vi "0x52.vi"(8 "error in":errorcluster, 10 "NTable":i32, 11 "paramUnicorn":T1={"conParam"={"ReadIntParam"=TRUE, "ReadDescrParam"=FALSE, "ReadFloatParam"=TRUE, "debug"=FALSE, "ReadJSON"=TRUE, "IP_address"="192.168.1.216", "N_attempts"=3, "type_con"=enum."TCP", "MB_address"=1, "VISA"="COM1", "connection ID"=refnum, "nameDevices"="", "timeout"=3000, "port"=2000, "type_version"="0F0C0001", "baud_rate"=115200, "VersionControl"=TRUE, "TCP_conn"=TRUE, "WindowSize"=700}, "Param"={"NumParam"={"NTelem"=201, "NInt"=16, "NFloat"=10, "NTable"=2}, "ParamInt"=[{"ID"="Режим работы", "Num"=0, "Name"="", "Type"="", "Enum"="", "Desc"="", "Unit"="", "Access"="", "FormatStr"="", "Min"=0, "Max"=0}, {"ID"="", "Num"=0, "Name"="", "Type"="", "Enum"="", "Desc"="", "Unit"="", "Access"="", "FormatStr"="", "Min"=0, "Max"=0}, {"ID"="", "Num"=0, "Name"="", "Type"="", "Enum"="", "Desc"="", "Unit"="", "Access"="", "FormatStr"="", "Min"=0, "Max"=0}, {"ID"="", "Num"=0, "Name"="", "Type"="", "Enum"="", "Desc"="", "Unit"="", "Access"="", "FormatStr"="", "Min"=0, "Max"=0}, {"ID"="", "Num"=0, "Name"="", "Type"="", "Enum"="", "Desc"="", "Unit"="", "Access"="", "FormatStr"="", "Min"=0, "Max"=0}, {"ID"="", "Num"=0, "Name"="", "Type"="", "Enum"="", "Desc"="", "Unit"="", "Access"="", "FormatStr"="", "Min"=0, "Max"=0}, {"ID"="ModeWork", "Num"=0, "Name"="", "Type"="", "Enum"="", "Desc"="", "Unit"="", "Access"="", "FormatStr"="", "Min"=0, "Max"=0}], "Telemetry"=[], "Table"=[], "ParamFloat"=[]}}) -> (0 "error out":errorcluster, 1 "ArrayFract32":fxp<+/-,32,1>[](array[numeric]), 2 "Table1D":sgl[](array[numeric]), 3 "paramUnicorn 2":T1={"conParam"={"ReadIntParam"=TRUE, "ReadDescrParam"=FALSE, "ReadFloatParam"=TRUE, "debug"=FALSE, "ReadJSON"=TRUE, "IP_address"="192.168.1.216", "N_attempts"=3, "type_con"=enum."TCP", "MB_address"=1, "VISA"="COM1", "connection ID"=refnum, "nameDevices"="", "timeout"=3000, "port"=2000, "type_version"="0F0C0001", "baud_rate"=115200, "VersionControl"=TRUE, "TCP_conn"=TRUE, "WindowSize"=700}, "Param"={"NumParam"={"NTelem"=201, "NInt"=16, "NFloat"=10, "NTable"=2}, "ParamInt"=[{"ID"="Режим работы", "Num"=0, "Name"="", "Type"="", "Enum"="", "Desc"="", "Unit"="", "Access"="", "FormatStr"="", "Min"=0, "Max"=0}, {"ID"="", "Num"=0, "Name"="", "Type"="", "Enum"="", "Desc"="", "Unit"="", "Access"="", "FormatStr"="", "Min"=0, "Max"=0}, {"ID"="", "Num"=0, "Name"="", "Type"="", "Enum"="", "Desc"="", "Unit"="", "Access"="", "FormatStr"="", "Min"=0, "Max"=0}, {"ID"="", "Num"=0, "Name"="", "Type"="", "Enum"="", "Desc"="", "Unit"="", "Access"="", "FormatStr"="", "Min"=0, "Max"=0}, {"ID"="", "Num"=0, "Name"="", "Type"="", "Enum"="", "Desc"="", "Unit"="", "Access"="", "FormatStr"="", "Min"=0, "Max"=0}, {"ID"="", "Num"=0, "Name"="", "Type"="", "Enum"="", "Desc"="", "Unit"="", "Access"="", "FormatStr"="", "Min"=0, "Max"=0}, {"ID"="ModeWork", "Num"=0, "Name"="", "Type"="", "Enum"="", "Desc"="", "Unit"="", "Access"="", "FormatStr"="", "Min"=0, "Max"=0}], "Telemetry"=[], "Table"=[], "ParamFloat"=[]}})   [LabVIEW 2017, in "LV_Unicorn.lvlib"]
uses:
  LV_Unicorn.lvlib
  Control/unicorn_Param.ctl
  Control/unicorn_conn.ctl
  Control/unicorn_JSON.ctl
  Control/unicorn_ParamInt.ctl
  Control/unicorn_Telemetry.ctl
  Control/unicorn_Table.ctl
  Control/unicorn_ParamFloat.ctl
panel:
  in  "Stop":bool
  out "Считывание табличных данных":u8(slide) scale=0.0..100.0
  out "Parameters":T8 {"Шаг по данным в словах" min=0 step=4; "Размер поля (слова) в байтах" min=0 step=4; "Размер записываемых данных в байтах" min=0 step=4}
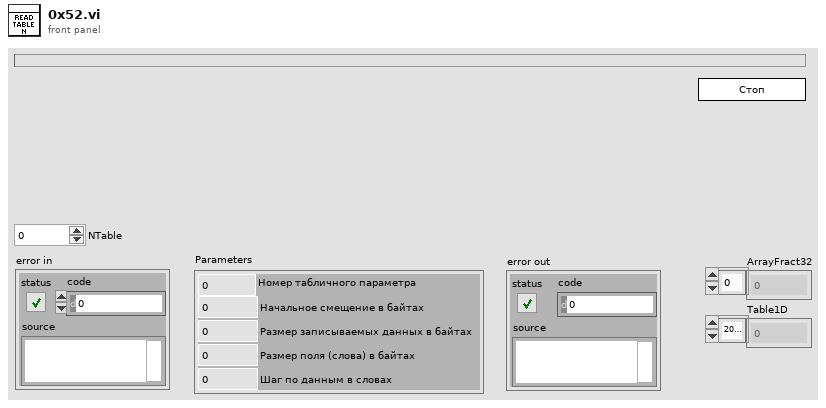
[diagram p1: front panel]
types:
  T1 = typedef "LV_Unicorn.lvlib/unicorn_Param.ctl" = cluster{"conParam":T2, "Param":T3}
  T2 = typedef "LV_Unicorn.lvlib/unicorn_conn.ctl" = cluster{"ReadIntParam":bool, "ReadDescrParam":bool, "ReadFloatParam":bool, "debug":bool, "ReadJSON":bool, "IP_address":string, "N_attempts":i32, "type_con":enum16{"Serial", "TCP"}, "MB_address":i32, "VISA":refnum<visa-resource-name>, "connection ID":refnum<k5>, "nameDevices":string, "timeout":i32, "port":u16, "type_version":string, "baud_rate":u32, "VersionControl":bool, "TCP_conn":bool, "WindowSize":i32}
  T3 = typedef "LV_Unicorn.lvlib/unicorn_JSON.ctl" = cluster{"NumParam":cluster{"NTelem":i32, "NInt":i32, "NFloat":i32, "NTable":i32}, "ParamInt":T4, "Telemetry":T5, "Table":T6, "ParamFloat":T7}
  T4 = typedef "LV_Unicorn.lvlib/unicorn_ParamInt.ctl" = cluster{"ID":string, "Num":i32, "Name":string, "Type":string, "Enum":string, "Desc":string, "Unit":string, "Access":string, "FormatStr":string, "Min":i32, "Max":i32}[]
  T5 = typedef "LV_Unicorn.lvlib/unicorn_Telemetry.ctl" = cluster{"ID":string, "Num":i32, "Name":string, "Desc":string, "Unit":string, "FormatStr":string, "Min":i32, "Max":i32}[]
  T6 = typedef "LV_Unicorn.lvlib/unicorn_Table.ctl" = cluster{"Num":i32, "Access":string, "ColumnCount":i32, "NeedParamPrepare":bool, "Columns":cluster{"Column":i32, "Desc":string, "Name":string}[], "DataType":string, "FormatStr":string, "ID":string, "Name":string, "RowCount":i32, "Rows":cluster{"Desc":string, "ID":string, "Max":i32, "Min":i32, "Name":string, "Row":i32, "Unit":string}[], "Type":string}[]
  T7 = typedef "LV_Unicorn.lvlib/unicorn_ParamFloat.ctl" = cluster{"ID":string, "Num":i32, "Name":string, "Type":string, "Enum":string, "Desc":string, "Unit":string, "Access":string, "FormatStr":string, "Min":sgl, "Max":sgl}[]
  T8 = cluster{"Начальное смещение в байтах":i32, "Номер табличного параметра":i32, "Размер записываемых данных в байтах":i32, "Размер поля (слова) в байтах":i32, "Шаг по данным в словах":i32}
  T9 = cluster{"Num":i32, "Access":string, "ColumnCount":i32, "NeedParamPrepare":bool, "Columns":cluster{"Column":i32, "Desc":string, "Name":string}[], "DataType":string, "FormatStr":string, "ID":string, "Name":string, "RowCount":i32, "Rows":cluster{"Desc":string, "ID":string, "Max":i32, "Min":i32, "Name":string, "Row":i32, "Unit":string}[], "Type":string}
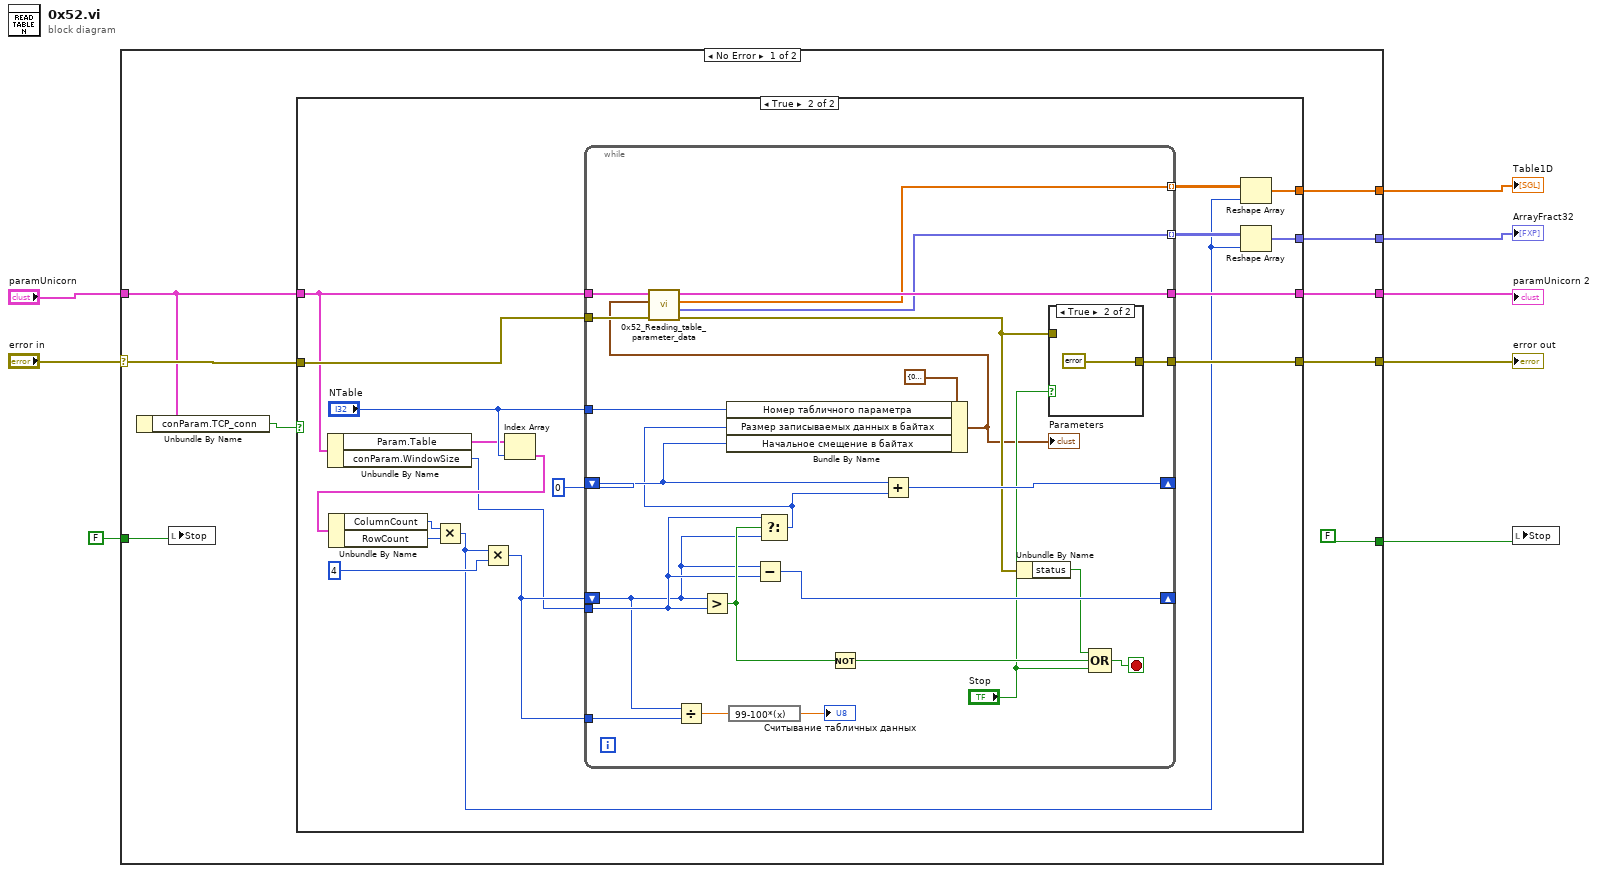
[diagram p0: block diagram]
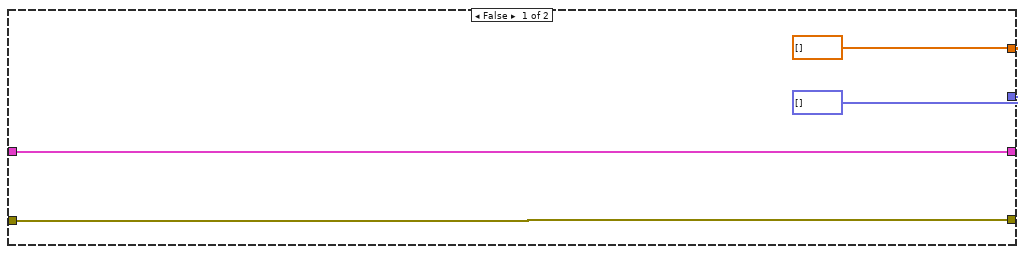
[diagram p2: hidden frame]
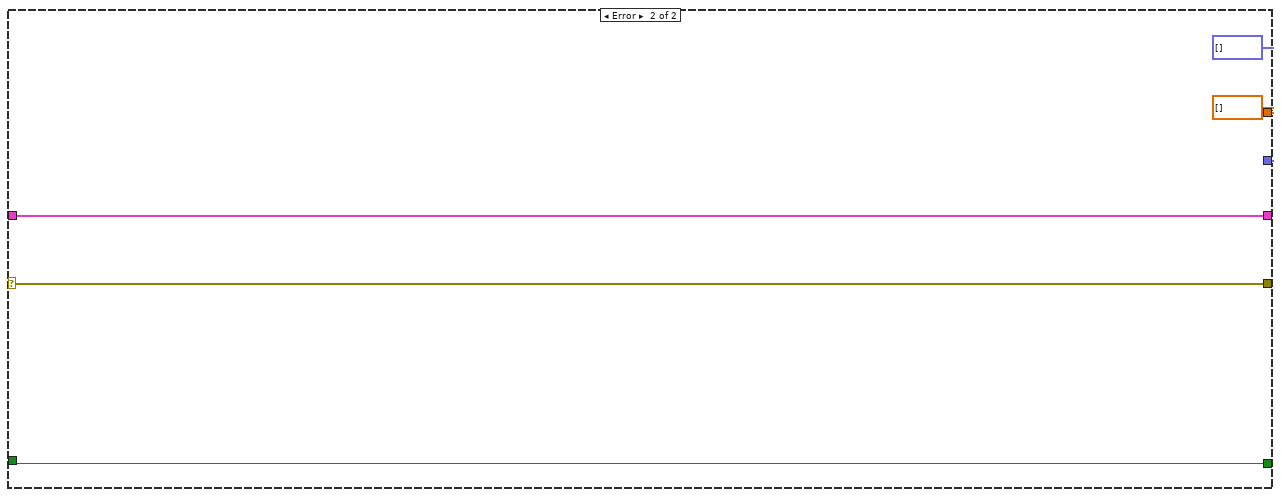
[diagram p4: hidden frame]
diagram:
  n1 = case shown="No Error" "error in" {
    selector: "error in" -> [w14 w70]
    tunnel: [w17 sgl[] []] -> w8
    tunnel: "paramUnicorn" -> [w12 w69]
    tunnel: [w16 w70] -> w7
    tunnel: [w15 w69] -> w3
    tunnel: [w13 fxp<+/-,32,1>[] [] ("ArrayFract32")] -> w5
    tunnel: FALSE ("Stop") -> [w10 w66]
    tunnel: [FALSE ("Stop") w66] -> w1
    frame No Error {
      n2 = Unbundle By Name(w12) -> ("conParam.TCP_conn"=w11:bool)
      n3 = local write "Stop"(w10) -> ()
      n4 = case shown="True" w11 {
        tunnel: [sgl[] [] w27] -> w17
        tunnel: [w18 w29] -> w16
        tunnel: [w19 w37] -> w15
        tunnel: w14 -> [w18 w36]
        tunnel: [fxp<+/-,32,1>[] [] ("ArrayFract32") w25] -> w13
        tunnel: w12 -> [w19 w33]
        frame False {
        }
        frame True {
          n5 = Unbundle By Name(w33) -> ("Param.Table"=w22:T6, "conParam.WindowSize"=w23:i32)
          n6 = Index Array(array=w22, index="NTable") -> (element=w32:T9)
          n7 = Unbundle By Name(w32) -> ("ColumnCount"=w31:i32, "RowCount"=w30:i32)
          n8 = Multiply(x=w31, y=w30) -> (x*y=w24:i32)
          n9 = Multiply(x=w24, y=4) -> (x*y=w35:i32)
          n10 = while {
            tunnel: w33 -> [w52]
            tunnel: w36 -> [w63]
            shift-right: [w62] -> _
            shift-left: w35 -> [w42]
            shift-right: [w59] -> _
            shift-left: 0 ("y") -> [w61]
            tunnel: "NTable" -> [w57]
            tunnel: [w48] -> w29
            tunnel: [w56] -> w37
            tunnel: w23 -> [w54]
            tunnel: w35 -> [w41]
            tunnel: [w45] -> w28 mode=indexing
            tunnel: [w44] -> w26 mode=indexing
            stop <- w50 stop-if-true
            n11 = Divide(x=w42, y=w41) -> (x/y=w40:dbl)
            n12 = Greater?(x=w42, y=w54) -> (0:w58:bool)
            n13 = expression code="99-100*(x)"(w40) -> (→"Считывание табличных данных":dbl)
            n14 = Subtract(x=w42, y=w54) -> (x-y=w62:i32)
            n15 = Select(t=w54, s=w58, f=w42) -> (s? t:f=w60:i32)
            n16 = Bundle By Name(cluster=T8 {"Начальное смещение в байтах"=0, "Номер табличного параметра"=0, "Размер записываемых данных в байтах"=0, "Размер поля (слова) в байтах"=4, "Шаг по данным в словах"=0} ("Cluster 3"), "Номер табличного параметра"=w57, "Размер записываемых данных в байтах"=w60, "Начальное смещение в байтах"=w61) -> (w43:T8)
            "Parameters" <- w43
            n17 = call "0x52_Reading_table_parameter_data.vi"("error in"=w63, "Param"=w43, "paramUnicorn in"=w52) -> ("error out"=w47:errorcluster, "ArrayFract32"=w44:fxp<+/-,32,1>[], "ArrayFloat"=w45:sgl[], "paramUnicorn"=w56:T1)  [unwired: 5 in]
            n18 = Not(x=w58) -> (.not. x?=w51:bool)
            n19 = Add(x=w61, y=w60) -> (x+y=w59:i32)
            n20 = Unbundle By Name(w47) -> ("status"=w49:bool)
            n21 = case shown="True" "Stop" {
              tunnel: [w64 errorcluster {"status"=TRUE, "code"=0, "source"="Пользователь остановил считывание таблицы."} ("error out")] -> w48
              tunnel: w47 -> [w64 _]
              frame False {
              }
              frame True {
              }
            }
            n22 = Compound Arithmetic op=OR(w49, w51, "Stop") -> (w50:bool)
          }
          n23 = Reshape Array(w28, w24) -> (w27:sgl[])
          n24 = Reshape Array(w26, w24) -> (w25:fxp<+/-,32,1>[])
        }
      }
    }
    frame Error {
    }
  }
  "Table1D" <- w8
  "error out" <- w7
  "ArrayFract32" <- w5
  "paramUnicorn 2" <- w3
  n25 = local write "Stop"(w1) -> ()
